vi "ASI_move_serial.vi"(4 "Position/distance (um)":dbl, 5 "error in":errorcluster, 6 "Relative?":bool, 7 "Axis":u16(ring)=2 items=["X", "Y", "Z"], 8 "VISA resource name":refnum<visa-resource-name>) -> (0 "error out":errorcluster, 3 "VISA resource name out":refnum<visa-resource-name>)   [LabVIEW 2018]
panel:
  out "Number of cycles":i32
  out "read buffer after STATUS":string
  out "Number of Bytes at Serial Port":u32
  out "read buffer after MOVE":string
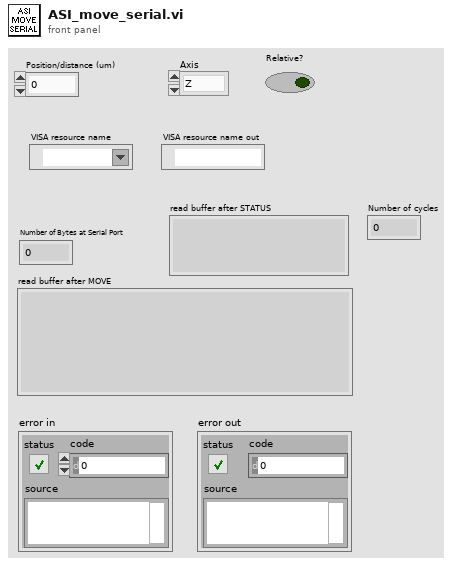
[diagram p1: front panel]
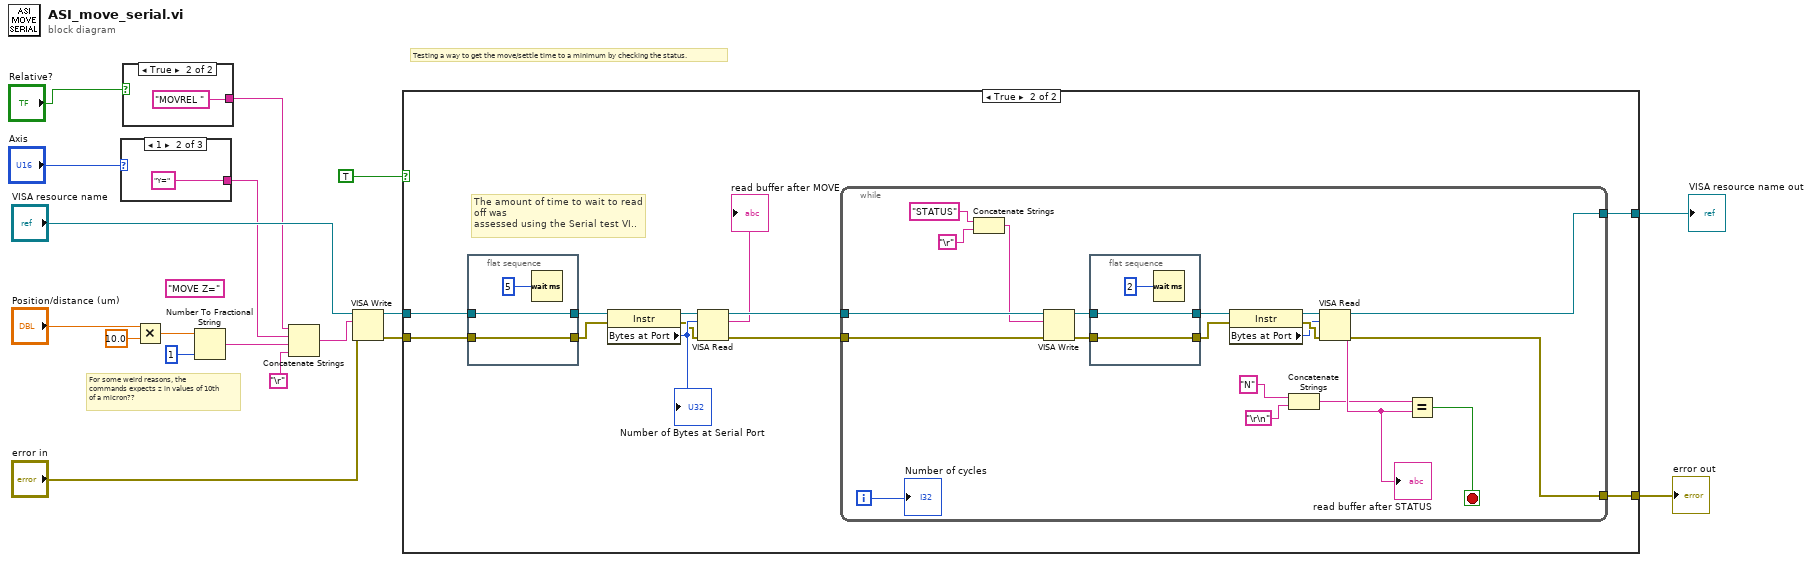
[diagram p0: block diagram]
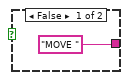
[diagram p2: hidden frame]
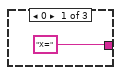
[diagram p3: hidden frame]
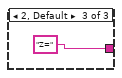
[diagram p4: hidden frame]
diagram:
  (unwired) "MOVE Z=" ("string")
  # "Testing a way to get the move/settle time to a minimum by checking the status."
  # "For some weird reasons, the \ncommands expects z in values of 10th \nof a micron??"
  n1 = case shown="1" "Axis" {
    tunnel: ["X=" "Y=" "Z="] -> w2
    frame 0 {
    }
    frame 1 {
    }
    frame 2, Default {
    }
  }
  n2 = case shown="True" "Relative?" {
    tunnel: ["MOVE " "MOVREL "] -> w3
    frame False {
    }
    frame True {
    }
  }
  n3 = Multiply(x="Position/distance (um)", y=10.0) -> (x*y=w7:dbl)
  n4 = Number To Fractional String(number=w7, precision (6)=i16 1) -> (F-format string=w9:string)  [unwired: 2 in]
  n5 = Concatenate Strings(w3, w2, w9, "\r") -> (w18:string)
  n6 = VISA Write(VISA resource name="VISA resource name", write buffer=w18, error in (no error)="error in") -> (VISA resource name out=w17:refnum<visa-resource-name>, error out=w14:errorcluster)  [unwired: 1 out]
  n7 = case shown="True" TRUE {
    tunnel: w17 -> [w25 w37]
    tunnel: w14 -> [w24 w36]
    tunnel: [w24 w32] -> w13
    tunnel: [w25 w33] -> w12
    frame False {
    }
    frame True {
      # "The amount of time to wait to read off was \nassessed using the Serial test VI.."
      n8 = flat-sequence {
        tunnel: [w40] -> w28
        tunnel: w37 -> [w40]
        tunnel: [w38] -> w27
        tunnel: w36 -> [w38]
        frame #0 {
          n9 = Wait (ms)(milliseconds to wait=u32 5) -> ()  [unwired: 1 out]
        }
      }
      n10 = property class="Instr"(reference=w28, error in=w27) -> (reference out=w31:refnum<visa-resource-name>, error out=w26:errorcluster, "Bytes at Port"=w30:u32)
      "Number of Bytes at Serial Port" <- w30
      n11 = VISA Read(VISA resource name=w31, byte count=w30, error in (no error)=w26) -> (VISA resource name out=w35:refnum<visa-resource-name>, read buffer=→"read buffer after MOVE":string, error out=w34:errorcluster)  [unwired: 1 out]
      n12 = while {
        tunnel: w35 -> [w60]
        tunnel: w34 -> [w59]
        tunnel: [w49] -> w33
        tunnel: [w48] -> w32
        i -> [w41]
        stop <- w50 stop-if-true
        n13 = Concatenate Strings("STATUS" ("write buffer"), "\r") -> (w43:string)
        n14 = VISA Write(VISA resource name=w60, write buffer=w43, error in (no error)=w59) -> (VISA resource name out=w53:refnum<visa-resource-name>, error out=w52:errorcluster)  [unwired: 1 out]
        n15 = flat-sequence {
          tunnel: [w63] -> w56
          tunnel: w53 -> [w63]
          tunnel: [w61] -> w57
          tunnel: w52 -> [w61]
          frame #0 {
            n16 = Wait (ms)(milliseconds to wait=u32 2) -> ()  [unwired: 1 out]
          }
        }
        n17 = property class="Instr"(reference=w56, error in=w57) -> (reference out=w54:refnum<visa-resource-name>, error out=w58:errorcluster, "Bytes at Port"=w55:u32)
        n18 = Concatenate Strings("N" ("x"), "\r\n") -> (w46:string)
        n19 = VISA Read(VISA resource name=w54, byte count=w55, error in (no error)=w58) -> (VISA resource name out=w49:refnum<visa-resource-name>, read buffer=w51:string, error out=w48:errorcluster)  [unwired: 1 out]
        "read buffer after STATUS" <- w51
        n20 = Equal?(x=w46, y=w51) -> (x = y?=w50:bool)
        "Number of cycles" <- w41
      }
    }
  }
  "error out" <- w13
  "VISA resource name out" <- w12
